vi "FTP_readmoviefile.vi"(0 "URL":string="192.168.1.101", 2 "Movie name":string, 3 "error in (no error)":errorcluster, 4 "local path":path=path "/Users/crogers/Desktop") -> (5 "Movie":path, 6 "Text":path, 7 "error out":errorcluster)   [LabVIEW 2015]
uses:
  <vilib>/FTP/NI_FTP.lvlib
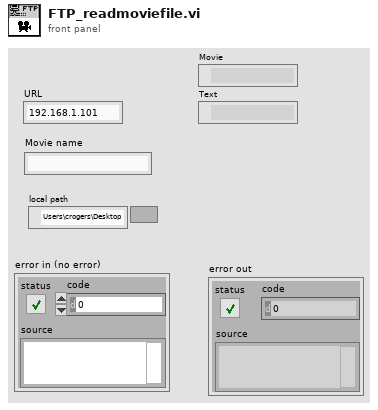
[diagram p1: front panel]
types:
  T1 = cluster{"Storage Dir":string, "Connection Information:":string}
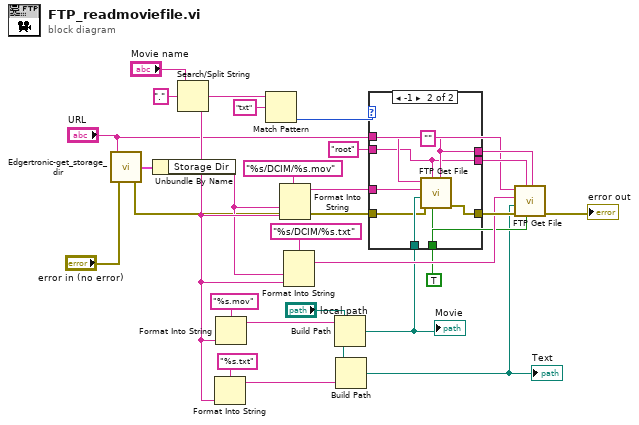
[diagram p0: block diagram]
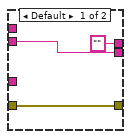
[diagram p2: hidden frame]
diagram:
  w19 = TRUE ("binary (F)")
  n1 = call "Edgertronic-get_storage_dir.vi"("error in (no error)"="error in (no error)", "URL"="URL") -> ("error out"=w3:errorcluster, "Storage Dir:"=w9:T1)  [unwired: 2 in]
  n2 = Unbundle By Name(w9) -> ("Storage Dir"=w8:string)
  n3 = Search/Split String(string="Movie name", search string/char (-)=".") -> (substring before match=w16:string, match + rest of string=w6:string)  [unwired: 1 in, 1 out]
  n4 = Format Into String(format string="%s.txt" ("remote path"), w16) -> (resulting string=w12:string)  [unwired: 2 in, 1 out]
  n5 = Format Into String(format string="%s.mov" ("remote path"), w16) -> (resulting string=w15:string)  [unwired: 2 in, 1 out]
  n6 = Match Pattern(string=w6, regular expression="txt") -> (offset past match=w2:i32)  [unwired: 1 in, 3 out]
  n7 = Format Into String(format string="%s/DCIM/%s.mov" ("remote path"), w8, w16) -> (resulting string=w25:string)  [unwired: 2 in, 1 out]
  n8 = Format Into String(format string="%s/DCIM/%s.txt" ("remote path"), w8, w16) -> (resulting string=w20:string)  [unwired: 2 in, 1 out]
  n9 = Build Path(base path="local path", name or relative path=w15) -> (appended path=w14:path)
  "Movie" <- w14
  n10 = Build Path(base path="local path", name or relative path=w12) -> (appended path=w11:path)
  "Text" <- w11
  n11 = case shown="-1" w2 {
    tunnel: w25 -> [_ w39]
    tunnel: [w29 w38] -> w24
    tunnel: [w31 w33] -> w23
    tunnel: ["" ("password") w37] -> w22
    tunnel: w19 -> [_ w36]
    tunnel: w14 -> [_ w35]
    tunnel: "URL" -> [_ w34]
    tunnel: "root" ("user") -> [w31 w33]
    tunnel: w3 -> [w29 w32]
    frame Default {
    }
    frame -1 {
      w37 = "" ("password")
      n12 = call <vilib>:"FTP Get File.vi"("password"=w37, "binary (F)"=w36, "user"=w33, "error in (no error)"=w32, "local path"=w35, "remote path"=w39, "host"=w34) -> ("error out"=w38:errorcluster)  [unwired: 3 in, 1 out]
    }
  }
  n13 = call <vilib>:"FTP Get File.vi"("password"=w22, "binary (F)"=w19, "user"=w23, "error in (no error)"=w24, "local path"=w11, "remote path"=w20, "host"="URL") -> ("error out"=→"error out":errorcluster)  [unwired: 3 in, 1 out]
